vi "cwlaserClose.vi"   [LabVIEW 2017]
uses:
  globalDevices.vi
types:
  T1 = cluster{"serialPort":refnum<visa-resource-name>, "error":errorcluster, "power (mW)":dbl, "wavelength (nm)":dbl, "type":string}[]
  T2 = cluster{"serialPort":refnum<visa-resource-name>, "error":errorcluster, "power (mW)":dbl, "wavelength (nm)":dbl, "type":string}
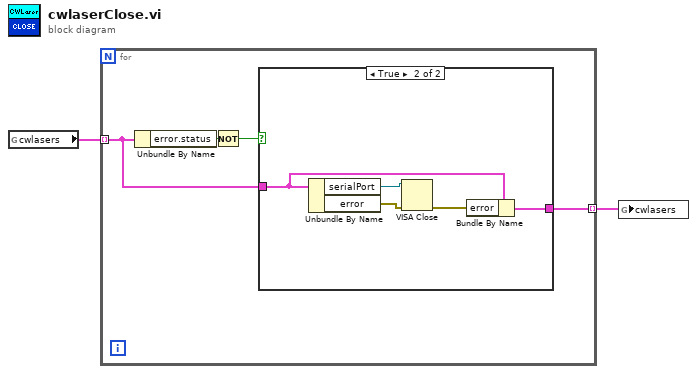
[diagram p0: block diagram]
diagram:
  n1 = global read "globalDevices.vi" "cwlasers"() -> (w2:T1)
  n2 = for {
    tunnel: w2 -> [w4] mode=indexing
    tunnel: [w3] -> w1 mode=indexing
    n3 = Unbundle By Name(w4) -> ("error.status"=w6:bool)
    n4 = Not(x=w6) -> (.not. x?=w5:bool)
    n5 = case shown="True" w5 {
      tunnel: w4 -> [w7 w10]
      tunnel: [w7 w8] -> w3
      frame False {
      }
      frame True {
        n6 = Unbundle By Name(w10) -> ("serialPort"=w12:refnum<visa-resource-name>, "error"=w11:errorcluster)
        n7 = VISA Close(VISA resource name=w12, error in (no error)=w11) -> (error out=w9:errorcluster)
        n8 = Bundle By Name(cluster=w10, "error"=w9) -> (w8:T2)
      }
    }
  }
  n9 = global write "globalDevices.vi" "cwlasers"(w1) -> ()
